vi "CameraManager.vi"(0 "Queue in":refnum<queue>, 2 "Save Setting":T5, 3 "Cluster In":T4={"Camera Mode"=FALSE, "顯示準星"=FALSE, "準星顏色"=65469}, 5 "Camera Manager Data":T3={"Camera Index"=0.0, "Exposure Time"=2800.0, "Image"=refnum, "Save Img Path"=path "C:/Users/MyUser/Pictures", "error out"={"status"=FALSE, "code"=0, "source"=""}, "Specific Parameter"={"Parameter Name"="", "Parameter Value"=""}, "Image Info"={"Height"=0.0, "Width"=0.0, "Channels"=0.0}}, 8 "Select Case":string, 11 "Pic Path":path=path "C:/Users/DavidHsu/OneDrive - PlayNitride/L0_230912/pic/key_pic/20x_2040_rf_k31l.bmp") -> (9 "save img path":path, 14 "Queue out":refnum<queue>, 16 "Initial Status":bool, 17 "Version Info":string, 18 "Camera Count(Output)":i32, 19 "Camera Manager Data Output":T3={"Camera Index"=0.0, "Exposure Time"=2800.0, "Image"=refnum, "Save Img Path"=path "C:/Users/MyUser/Pictures", "error out"={"status"=FALSE, "code"=0, "source"=""}, "Specific Parameter"={"Parameter Name"="", "Parameter Value"=""}, "Image Info"={"Height"=0.0, "Width"=0.0, "Channels"=0.0}})   [LabVIEW 2017, in "PlayNitrideCameraComponet1010_4.lvlib"]
uses:
  <userlib>/PlayNitrideCameraComponet1010_4/PlayNitrideCameraComponet1010_4.lvlib
  <vilib>/vision/Image Controls.llb/IMAQ Image.ctl
  <userlib>/PlayNitrideCameraComponet1010_4/cam_Global.vi
  <resource>/objmgr/IMAQImage.rc
panel:
  out "Camera Mode":bool
  out "Version":string
  in  "Image Info":T1
  out "Camera Count":i32
  out "Initial Success":bool
  out "Stop":bool
  # "中間內部變數 如果有需求可以拉出接口"
  # "Input"
  # "Output"
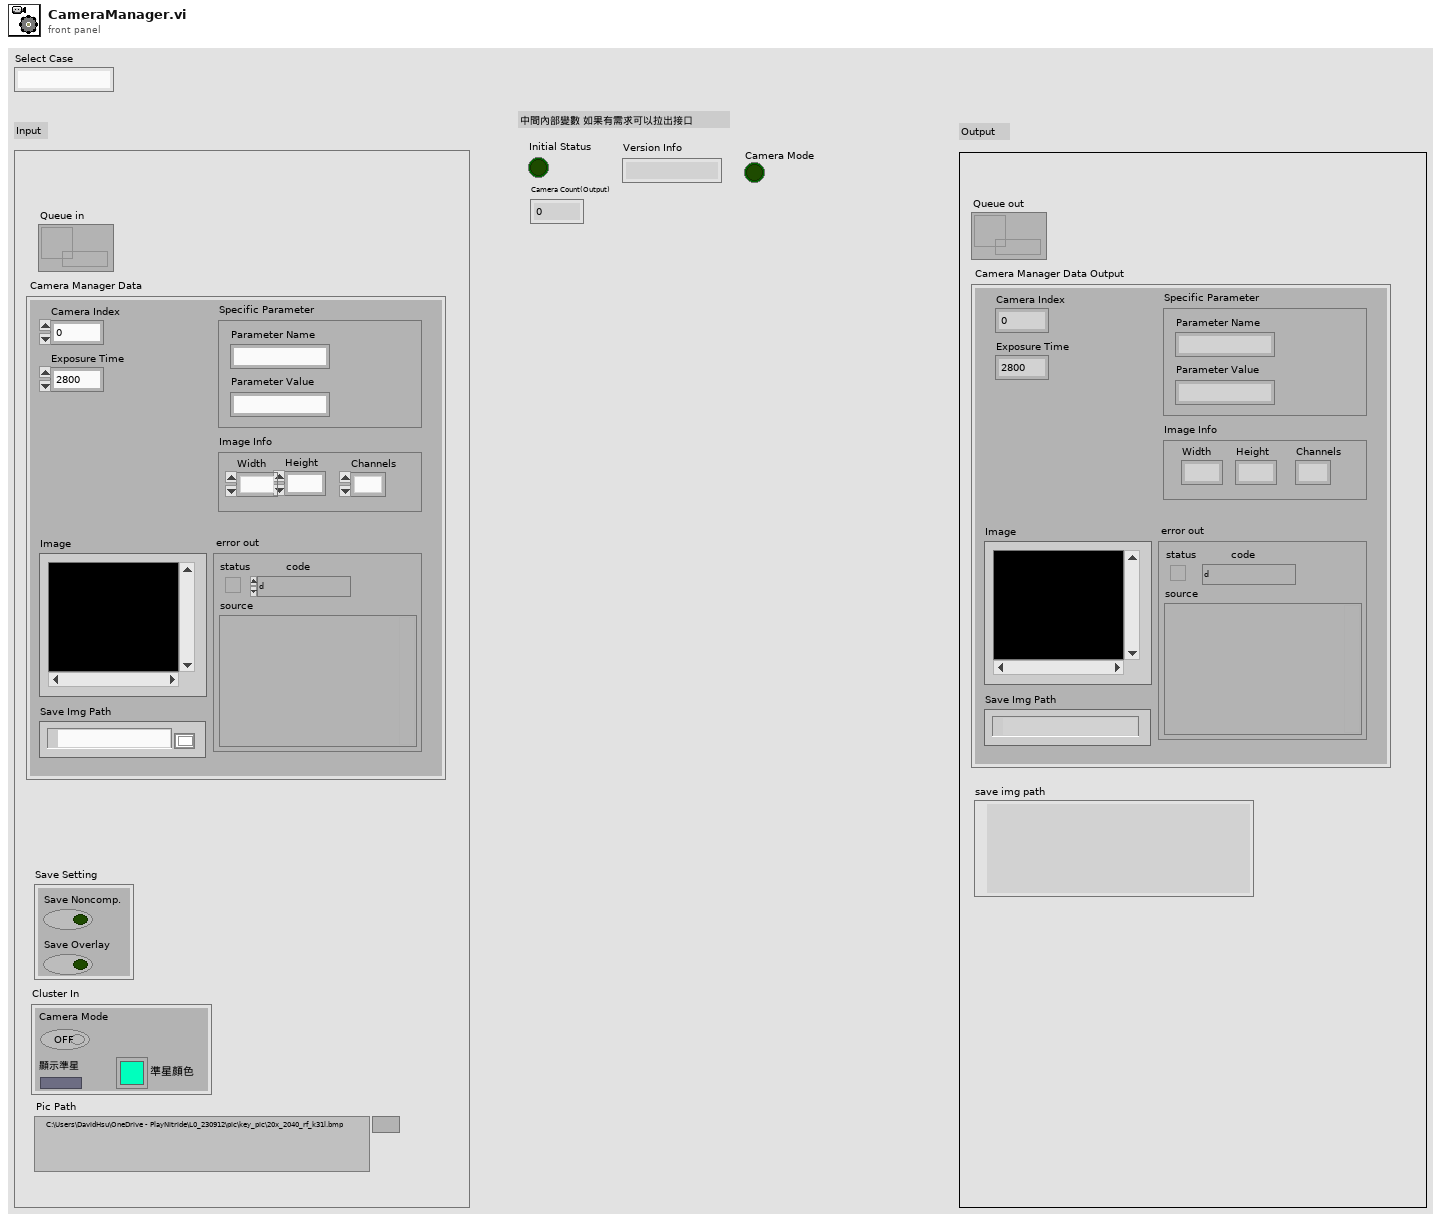
[diagram p1: front panel]
types:
  T1 = cluster{"Height":dbl, "Width":dbl, "Channels":dbl}
  T2 = typedef "IMAQ Image.ctl" = refnum<image>
  T3 = cluster{"Camera Index":dbl, "Exposure Time":dbl, "Image":T2, "Save Img Path":path, "error out":errorcluster, "Specific Parameter":cluster{"Parameter Name":string, "Parameter Value":string}, "Image Info":cluster{"Height":dbl, "Width":dbl, "Channels":dbl}}
  T4 = cluster{"Camera Mode":bool, "顯示準星":bool, "準星顏色":u32}
  T5 = cluster{"Save Noncomp.":bool, "Save Overlay":bool}
  T6 = typedef "Image Type" = u32
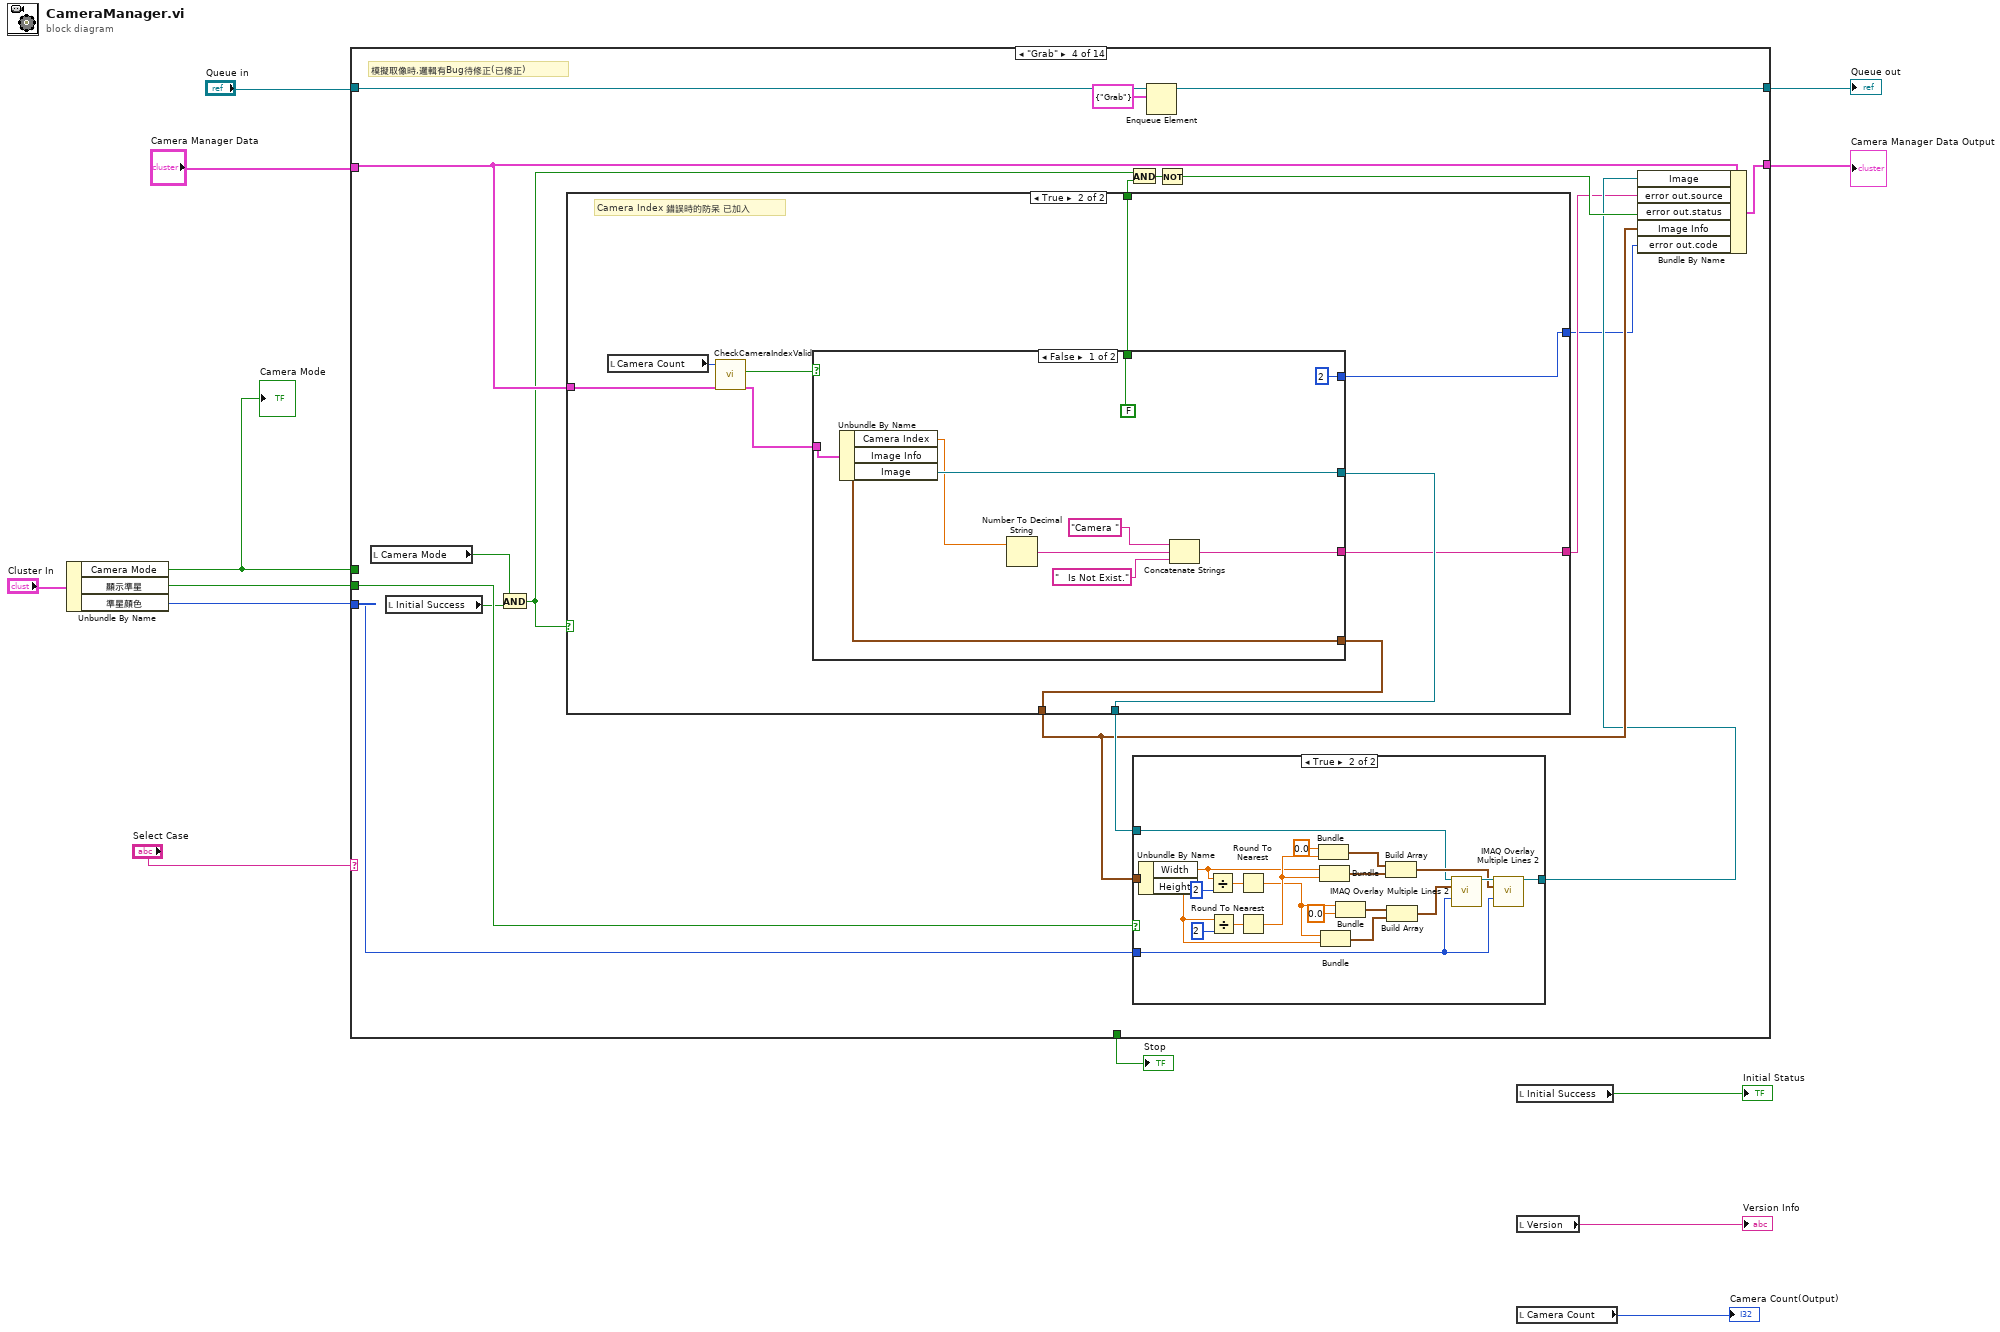
[diagram p0: block diagram]
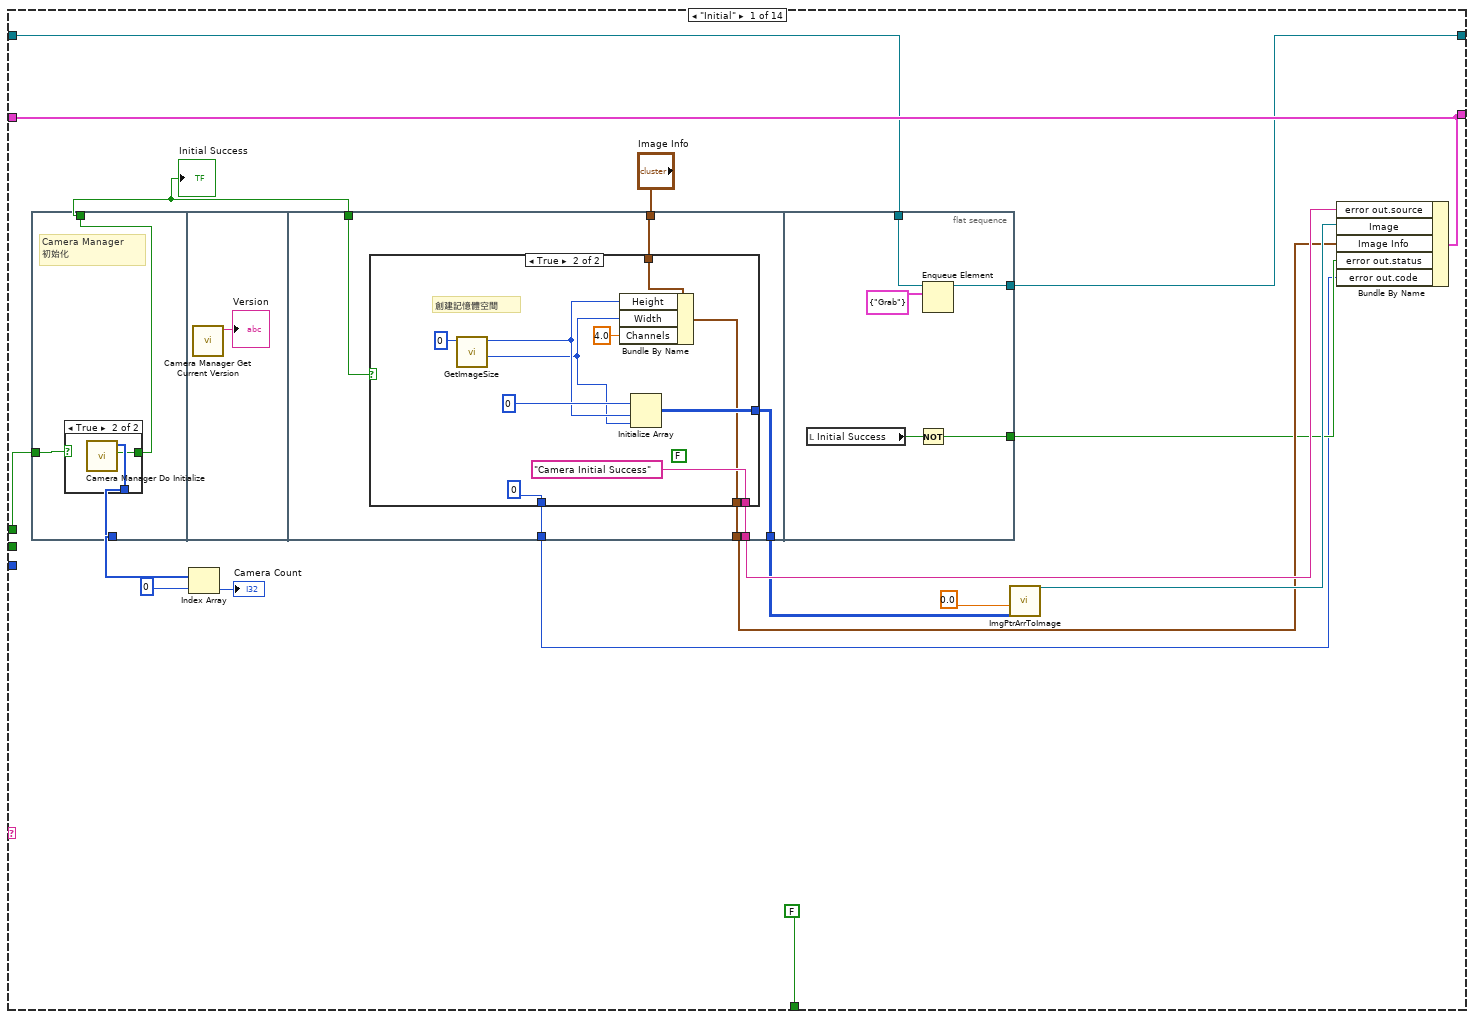
[diagram p2: hidden frame]
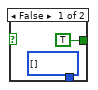
[diagram p3: hidden frame]
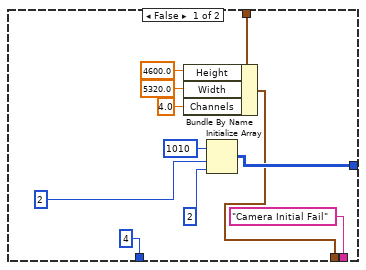
[diagram p4: hidden frame]
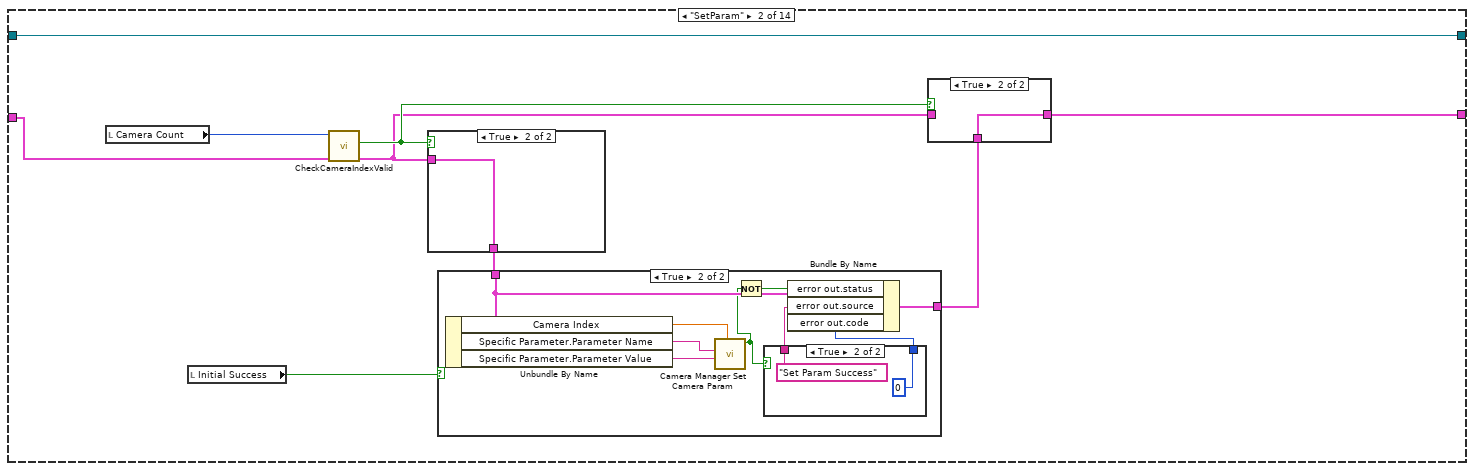
[diagram p5: hidden frame]
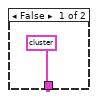
[diagram p7: hidden frame]
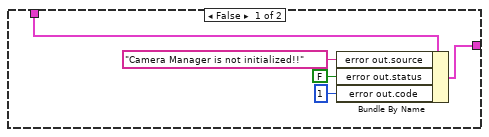
[diagram p8: hidden frame]
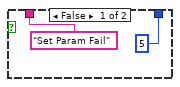
[diagram p9: hidden frame]
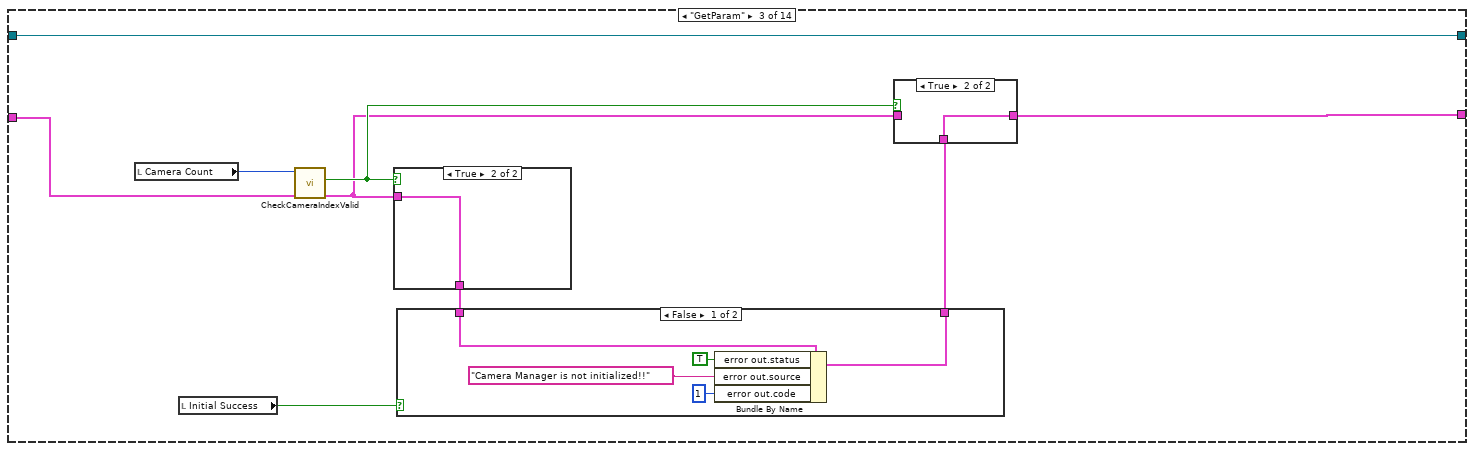
[diagram p10: hidden frame]
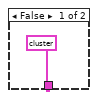
[diagram p12: hidden frame]
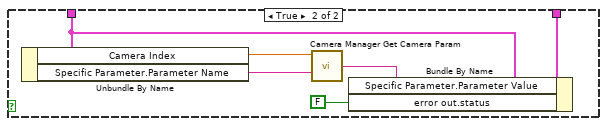
[diagram p13: hidden frame]
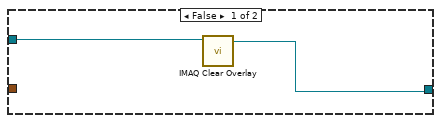
[diagram p14: hidden frame]
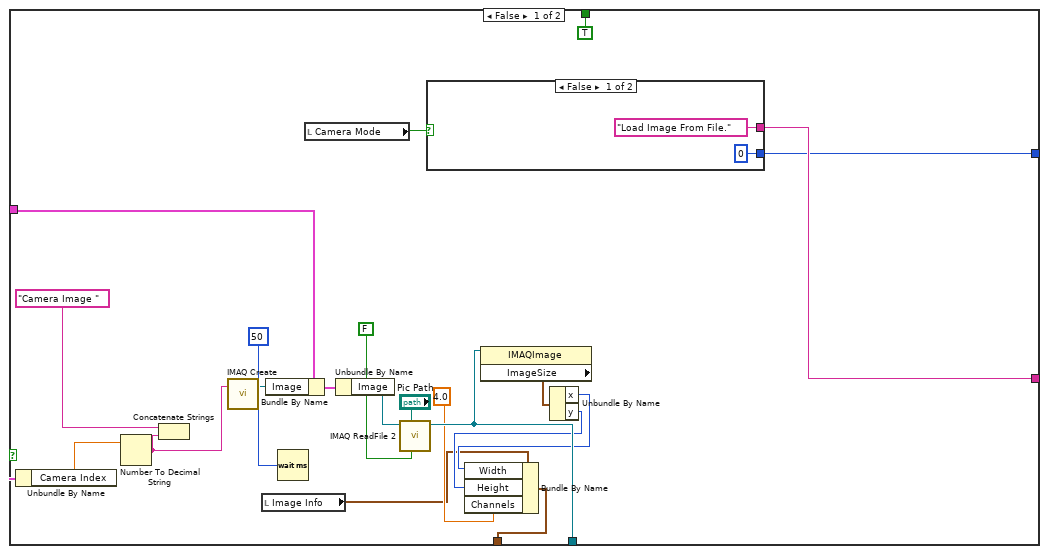
[diagram p15: hidden frame]
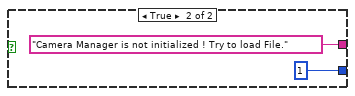
[diagram p16: hidden frame]
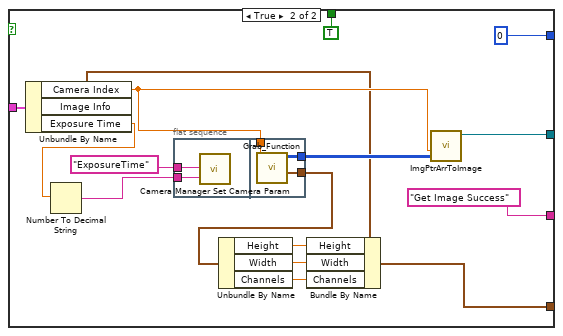
[diagram p17: hidden frame]
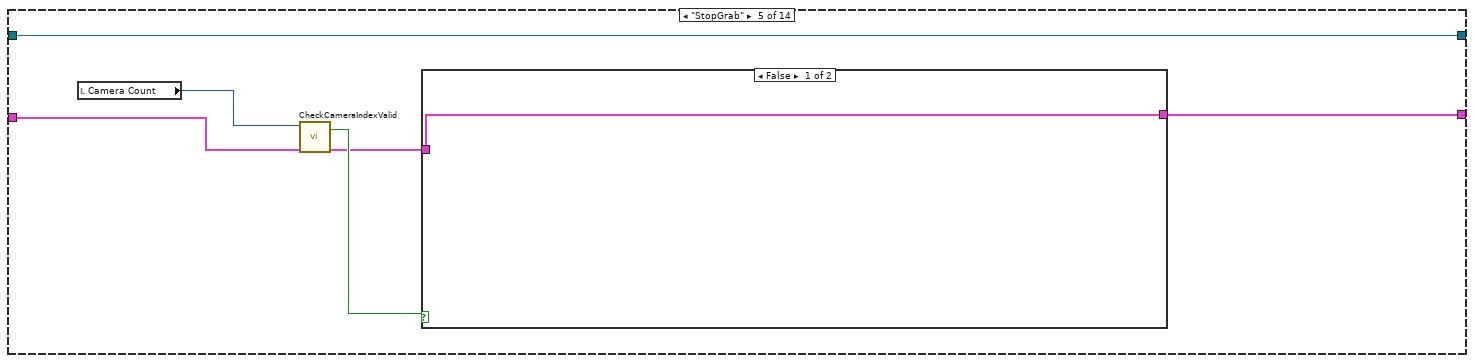
[diagram p18: hidden frame]
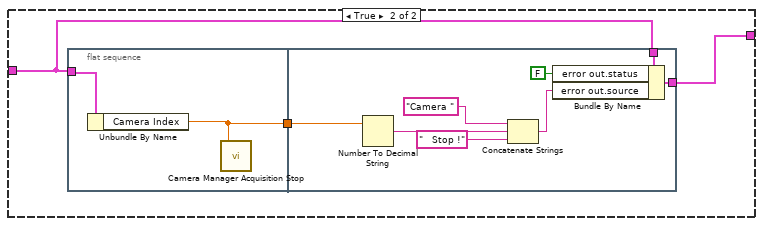
[diagram p19: hidden frame]
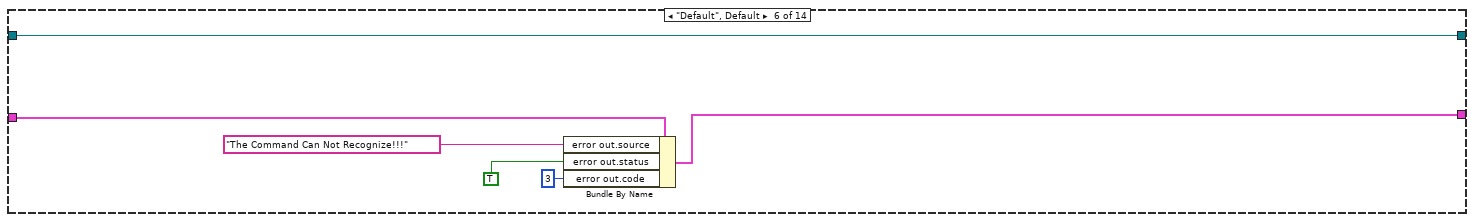
[diagram p20: hidden frame]
diagram:
  n1 = Unbundle By Name("Cluster In") -> ("Camera Mode"=w8:bool, "顯示準星"=w7:bool, "準星顏色"=w6:u32)
  "Camera Mode" <- w8
  n2 = case shown="\"Grab\"" "Select Case" {
    tunnel: "Queue in" -> [w18 w79 w110 w135 w237 w257 w277 w306 w337 w361 w368 w389 w400 w405]
    tunnel: [FALSE _ _ _ _ _ _ _ _ _ _ TRUE _ _] -> w13
    tunnel: [w17 w79 w110 w132 w237 w257 w277 w306 w337 w361 w368 w389 w400 w405] -> w11
    tunnel: [w28 w71 w105 w143 w232 w254 w258 w285 w310 w341 w366 w387 w397 w403] -> w4
    tunnel: "Camera Manager Data" -> [w28 w74 w107 w138 w233 w255 w258 w285 w310 w341 w367 w388 w398 w404]
    tunnel: w8 -> [w16 _ _ _ _ _ _ _ _ _ _ _ _ _]
    tunnel: w7 -> [_ _ _ w141 _ _ _ _ _ _ _ _ _ _]
    tunnel: w6 -> [_ _ _ w142 _ _ _ _ _ _ _ _ _ _]
    frame "Initial" {
      (unwired) FALSE
      n3 = flat-sequence {
        tunnel: [w31] -> w21
        tunnel: [w32] -> w30
        tunnel: w16 -> [w33]
        tunnel: w21 -> [w44]
        tunnel: [w43] -> w26
        tunnel: [w42] -> w27
        tunnel: [w41] -> w23
        tunnel: "Image Info" -> [w40]
        tunnel: [w39] -> w14
        tunnel: [w70] -> w22
        tunnel: w18 -> [w68]
        tunnel: [w67] -> w17
        frame #0 {
          # "Camera Manager \n初始化"
          n4 = case shown="True" w33 {
            tunnel: [i32[] [] ("CameraCount") w37] -> w32
            tunnel: [TRUE ("function return") w36] -> w31
            frame False {
            }
            frame True {
              n5 = call <userlib>:"Camera Manager Do Initialize.vi"() -> ("function return"=w36:bool, "CameraCount"=w37:i32[])  [unwired: 9 in, 1 out]
            }
          }
        }
        frame #1 {
          n6 = call <userlib>:"Camera Manager Get Current Version.vi"() -> ("function return"=→"Version":string)  [unwired: 10 in, 1 out]
        }
        frame #2 {
          n7 = case shown="True" w44 {
            tunnel: [w55 w64] -> w43
            tunnel: ["Camera Initial Fail" ("error out.source") "Camera Initial Success" ("error out.source")] -> w42
            tunnel: [w49 w60] -> w41
            tunnel: w40 -> [w50 w62]
            tunnel: [4 0] -> w39
            frame False {
              n8 = Bundle By Name(cluster=w50, "Height"=4600.0, "Width"=5320.0, "Channels"=4.0) -> (w49:T1)
              n9 = Initialize Array(u32 1010 ("element"), 2 ("dimension size"), 2 ("dimension size")) -> (w55:u32[][])
            }
            frame True {
              # "創建記憶體空間"
              n10 = call <userlib>:"GetImageSize.vi"("cameraId"=0) -> ("Width"=w57:i32, "Height"=w58:i32)  [unwired: 9 in]
              n11 = Bundle By Name(cluster=w62, "Height"=w58, "Width"=w57, "Channels"=4.0) -> (w60:T1)
              n12 = Initialize Array(u32 0 ("unsigned 32bit integer"), w58, w57) -> (w64:u32[][])
            }
          }
        }
        frame #3 {
          n13 = local read "Initial Success"() -> (w69:bool)
          n14 = Not(x=w69) -> (.not. x?=w70:bool)
          n15 = Enqueue Element(queue=w68, element=cluster{"State":string} {"State"="Grab"}) -> (queue out=w67:refnum<queue>)  [unwired: 2 in, 2 out]
        }
      }
      n16 = Index Array(array=w30, index=0) -> (element=→"Camera Count":i32)
      n17 = call <userlib>:"ImgPtrArrToImage.vi"("CameraIndex"=0.0, "Image Pixels (U32)"=w26) -> ("image out"=w25:T2)  [unwired: 8 in, 1 out]
      n18 = Bundle By Name(cluster=w28, "error out.source"=w27, "Image"=w25, "Image Info"=w23, "error out.status"=w22, "error out.code"=w14) -> ()  [unwired: 1 out]
      "Initial Success" <- w21
    }
    frame "SetParam" {
      n19 = local read "Camera Count"() -> (w75:i32)
      n20 = local read "Initial Success"() -> (w78:bool)
      n21 = call <userlib>:"CheckCameraIndexValid.vi"("Camera Manager Data"=w74, "CameraCount"=w75) -> ("Camera Manager Data Out"=w76:T3, "IsValidIndex"=w77:bool)  [unwired: 8 in]
      n22 = case shown="True" w77 {
        tunnel: [T3 {"Camera Index"=0.0, "Exposure Time"=0.0, "Image"=refnum, "Save Img Path"=path "", "error out"={"status"=FALSE, "code"=0, "source"=""}, "Specific Parameter"={"Parameter Name"="", "Parameter Value"=""}, "Image Info"={"Height"=0.0, "Width"=0.0, "Channels"=0.0}} ("Camera Manager Data Out") w83] -> w73
        tunnel: w76 -> [_ w83]
        frame False {
        }
        frame True {
        }
      }
      n23 = case shown="True" w78 {
        tunnel: w73 -> [w88 w96]
        tunnel: [w87 w97] -> w72
        frame False {
          n24 = Bundle By Name(cluster=w88, "error out.source"="Camera Manager is not initialized!!", "error out.status"=FALSE, "error out.code"=1) -> (w87:T3)
        }
        frame True {
          n25 = Unbundle By Name(w96) -> ("Camera Index"=w95:dbl, "Specific Parameter.Parameter Name"=w94:string, "Specific Parameter.Parameter Value"=w93:string)
          n26 = call <userlib>:"Camera Manager Set Camera Param.vi"("Value"=w93, "NodeName"=w94, "cameraId"=w95) -> ("function return"=w90:bool)  [unwired: 5 in, 3 out]
          n27 = Not(x=w90) -> (.not. x?=w89:bool)
          n28 = case shown="True" w90 {
            tunnel: ["Set Param Fail" ("error out.source") "Set Param Success" ("error out.source")] -> w92
            tunnel: [5 0] -> w91
            frame False {
            }
            frame True {
            }
          }
          n29 = Bundle By Name(cluster=w96, "error out.status"=w89, "error out.source"=w92, "error out.code"=w91) -> (w97:T3)
        }
      }
      n30 = case shown="True" w77 {
        tunnel: [w80 w81] -> w71
        tunnel: w72 -> [_ w81]
        tunnel: w76 -> [w80 _]
        frame False {
        }
        frame True {
        }
      }
    }
    frame "GetParam" {
      n31 = local read "Camera Count"() -> (w108:i32)
      n32 = local read "Initial Success"() -> (w109:bool)
      n33 = call <userlib>:"CheckCameraIndexValid.vi"("Camera Manager Data"=w107, "CameraCount"=w108) -> ("Camera Manager Data Out"=w102:T3, "IsValidIndex"=w103:bool)  [unwired: 8 in]
      n34 = case shown="True" w103 {
        tunnel: [T3 {"Camera Index"=0.0, "Exposure Time"=0.0, "Image"=refnum, "Save Img Path"=path "", "error out"={"status"=FALSE, "code"=0, "source"=""}, "Specific Parameter"={"Parameter Name"="", "Parameter Value"=""}, "Image Info"={"Height"=0.0, "Width"=0.0, "Channels"=0.0}} ("Camera Manager Data Out") w114] -> w106
        tunnel: w102 -> [_ w114]
        frame False {
        }
        frame True {
        }
      }
      n35 = case shown="False" w109 {
        tunnel: w106 -> [w119 w125]
        tunnel: [w118 w124] -> w104
        frame False {
          n36 = Bundle By Name(cluster=w119, "error out.status"=TRUE, "error out.source"="Camera Manager is not initialized!!", "error out.code"=1) -> (w118:T3)
        }
        frame True {
          n37 = Unbundle By Name(w125) -> ("Camera Index"=w120:dbl, "Specific Parameter.Parameter Name"=w121:string)
          n38 = call <userlib>:"Camera Manager Get Camera Param.vi"("NodeName"=w121, "cameraId"=w120) -> ("Value out"=w122:string)  [unwired: 7 in, 2 out]
          n39 = Bundle By Name(cluster=w125, "Specific Parameter.Parameter Value"=w122, "error out.status"=FALSE) -> (w124:T3)
        }
      }
      n40 = case shown="True" w103 {
        tunnel: [w111 w112] -> w105
        tunnel: w104 -> [_ w112]
        tunnel: w102 -> [w111 _]
        frame False {
        }
        frame True {
        }
      }
    }
    frame "Grab" {
      # "模擬取像時,邏輯有Bug待修正(已修正)"
      n41 = local read "Camera Mode"() -> (w134:bool)
      n42 = local read "Initial Success"() -> (w136:bool)
      n43 = And(x=w134, y=w136) -> (x .and. y?=w129:bool)
      n44 = case shown="True" w129 {
        tunnel: [w169 w195] -> w130
        tunnel: [w180 w197] -> w137
        tunnel: [w185 w196] -> w140
        tunnel: w138 -> [w174 w194]
        tunnel: [TRUE ("y") w193] -> w127
        tunnel: [w167 w192] -> w126
        frame False {
          n45 = Unbundle By Name(w174) -> ("Camera Index"=w173:dbl)
          n46 = Number To Decimal String(number=w173) -> (decimal integer string=w172:string)  [unwired: 1 in]
          n47 = Concatenate Strings("Camera Image " ("string"), w172) -> ()  [unwired: 1 out]
          n48 = call "IMAQ Create"("Image Name"=w172) -> ("New Image"=w176:T2)  [unwired: 4 in, 1 out]
          n49 = local read "Image Info"() -> (w179:T1)
          n50 = Bundle By Name(cluster=w174, "Image"=w176) -> (w178:T3)
          n51 = Wait (ms)(milliseconds to wait=u32 50) -> ()  [unwired: 1 out]
          n52 = local read "Camera Mode"() -> (w170:bool)
          n53 = Unbundle By Name(w178) -> ("Image"=w177:T2)
          n54 = call "IMAQ ReadFile 2"("Use File Path Image Type"=FALSE, "File Path"="Pic Path", "Image"=w177) -> ("Image Out"=w185:T2)  [unwired: 4 in, 4 out]
          n55 = case shown="False" w170 {
            tunnel: ["Load Image From File." ("error out.source") "Camera Manager is not initialized ! Try to load File." ("error out.source")] -> w169
            tunnel: [0 1] -> w167
            frame False {
            }
            frame True {
            }
          }
          n56 = property class="IMAQImage"(reference=w185) -> ("ImageSize"=w184:cluster{"x":i32, "y":i32})  [unwired: 1 in, 2 out]
          n57 = Unbundle By Name(w184) -> ("x"=w182:i32, "y"=w181:i32)
          n58 = Bundle By Name(cluster=w179, "Width"=w182, "Height"=w181, "Channels"=4.0) -> (w180:T1)
        }
        frame True {
          # "Camera Index 錯誤時的防呆 已加入"
          n59 = local read "Camera Count"() -> (w200:i32)
          n60 = call <userlib>:"CheckCameraIndexValid.vi"("Camera Manager Data"=w194, "CameraCount"=w200) -> ("Camera Manager Data Out"=w198:T3, "IsValidIndex"=w199:bool)  [unwired: 8 in]
          n61 = case shown="False" w199 {
            tunnel: w198 -> [w210 w217]
            tunnel: [w203 "Get Image Success" ("error out.source")] -> w195
            tunnel: [w206 w215] -> w197
            tunnel: [w205 w213] -> w196
            tunnel: [FALSE ("y") TRUE ("y")] -> w193
            tunnel: [2 0] -> w192
            frame False {
              n62 = Unbundle By Name(w210) -> ("Camera Index"=w202:dbl, "Image Info"=w206:T1, "Image"=w205:T2)
              n63 = Number To Decimal String(number=w202) -> (decimal integer string=w209:string)  [unwired: 1 in]
              n64 = Concatenate Strings("Camera " ("string"), w209, "   Is Not Exist." ("string")) -> (w203:string)
            }
            frame True {
              n65 = Unbundle By Name(w217) -> ("Camera Index"=w226:dbl, "Image Info"=w219:T1, "Exposure Time"=w214:dbl)
              n66 = Number To Decimal String(number=w214) -> (decimal integer string=w225:string)  [unwired: 1 in]
              n67 = flat-sequence {
                tunnel: "ExposureTime" ("NodeName") -> [w228]
                tunnel: w225 -> [w227]
                tunnel: [w231] -> w223
                tunnel: [w230] -> w224
                tunnel: w226 -> [w229]
                frame #0 {
                  n68 = call <userlib>:"Camera Manager Set Camera Param.vi"("Value"=w227, "NodeName"=w228) -> ()  [unwired: 6 in, 4 out]
                }
                frame #1 {
                  n69 = call <userlib>:"Grab_Function.vi"("cameraId"=w229) -> ("output cluster"=w231:T1, "imgPtr"=w230:i32[][])  [unwired: 7 in]
                }
              }
              n70 = Unbundle By Name(w223) -> ("Height"=w220:dbl, "Width"=w221:dbl, "Channels"=w222:dbl)
              n71 = Bundle By Name(cluster=w219, "Height"=w220, "Width"=w221, "Channels"=w222) -> (w215:T1)
              n72 = call <userlib>:"ImgPtrArrToImage.vi"("CameraIndex"=w226, "Image Pixels (U32)"=w224) -> ("image out"=w213:T2)  [unwired: 8 in, 1 out]
            }
          }
        }
      }
      n73 = And(x=w129, y=w127) -> (x .and. y?=w128:bool)
      n74 = case shown="True" w141 {
        tunnel: [w145 w165] -> w131
        tunnel: w137 -> [_ w155]
        tunnel: w140 -> [w144 w146]
        tunnel: w142 -> [_ w147]
        frame False {
          n75 = call "IMAQ Clear Overlay"("Image"=w144) -> ("Image Out"=w145:T2)  [unwired: 9 in, 1 out]
        }
        frame True {
          n76 = Unbundle By Name(w155) -> ("Width"=w161:dbl, "Height"=w148:dbl)
          n77 = Divide(x=w161, y=2) -> (x/y=w156:dbl)
          n78 = Divide(x=w148, y=2) -> (x/y=w157:dbl)
          n79 = Round To Nearest(number=w156) -> (nearest integer value=w162:dbl)
          n80 = Round To Nearest(number=w157) -> (nearest integer value=w164:dbl)
          n81 = Bundle("X"=0.0, w164) -> (w163:cluster{"X":dbl, dbl})  [unwired: 1 in]
          n82 = Bundle("Width"=w161, w164) -> (w160:cluster{"Width":dbl, dbl})  [unwired: 1 in]
          n83 = Bundle(w162, "Height"=w148) -> (w159:cluster{dbl, "Height":dbl})  [unwired: 1 in]
          n84 = Bundle(w162, "X"=0.0) -> (w158:cluster{dbl, "X":dbl})  [unwired: 1 in]
          n85 = Build Array(w163, w160) -> (w150:cluster{"Width":dbl, dbl}[])
          n86 = Build Array(w158, w159) -> (w149:cluster{dbl, "Height":dbl}[])
          n87 = call "IMAQ Overlay Multiple Lines 2"("Image"=w146, "Line End Points"=w149, "Color"=w147) -> ("Image Out"=w166:T2)  [unwired: 11 in, 1 out]
          n88 = call "IMAQ Overlay Multiple Lines 2"("Image"=w166, "Line End Points"=w150, "Color"=w147) -> ("Image Out"=w165:T2)  [unwired: 11 in, 1 out]
        }
      }
      n89 = Enqueue Element(queue=w135, element=cluster{"State":string} {"State"="Grab"}) -> (queue out=w132:refnum<queue>)  [unwired: 2 in, 2 out]
      n90 = Not(x=w128) -> (.not. x?=w139:bool)
      n91 = Bundle By Name(cluster=w138, "Image"=w131, "error out.source"=w130, "error out.status"=w139, "Image Info"=w137, "error out.code"=w126) -> (w143:T3)
    }
    frame "StopGrab" {
      n92 = local read "Camera Count"() -> (w236:i32)
      n93 = call <userlib>:"CheckCameraIndexValid.vi"("Camera Manager Data"=w233, "CameraCount"=w236) -> ("Camera Manager Data Out"=w234:T3, "IsValidIndex"=w235:bool)  [unwired: 8 in]
      n94 = case shown="False" w235 {
        tunnel: w234 -> [w238 w239]
        tunnel: [w238 w241] -> w232
        frame False {
        }
        frame True {
          n95 = flat-sequence {
            tunnel: w239 -> [w243]
            tunnel: [w242] -> w240
            tunnel: w239 -> [w249]
            tunnel: [w245] -> w241
            tunnel: w240 -> [w244]
            frame #0 {
              n96 = Unbundle By Name(w243) -> ("Camera Index"=w242:dbl)
              n97 = call <userlib>:"Camera Manager Acquisition Stop.vi"("cameraId"=w242) -> ()  [unwired: 10 in, 1 out]
            }
            frame #1 {
              n98 = Number To Decimal String(number=w244) -> (decimal integer string=w250:string)  [unwired: 1 in]
              n99 = Concatenate Strings("Camera " ("string"), w250, "   Stop !" ("string")) -> (w251:string)
              n100 = Bundle By Name(cluster=w249, "error out.status"=FALSE, "error out.source"=w251) -> (w245:T3)
            }
          }
        }
      }
    }
    frame "Default", Default {
      n101 = Bundle By Name(cluster=w255, "error out.source"="The Command Can Not Recognize!!!", "error out.status"=TRUE, "error out.code"=3) -> (w254:T3)
    }
    frame "Save Img" {
      # "這邊完全照抄 Kernel_Camera.vi 的內容"
      n102 = Unbundle By Name(w258) -> ("Save Img Path"=w272:path, "Image"=w265:T2)
      n103 = Get Date/Time In Seconds() -> (seconds since 1Jan1904=w271:timestamp)
      n104 = Unbundle By Name("Save Setting") -> ("Save Noncomp."=w262:bool, "Save Overlay"=w267:bool)
      n105 = Format Date/Time String(time format string (%c)="%Y%m%d_%H%M%S", seconds (now)=w271) -> (date/time string=w269:string)  [unwired: 1 in]
      n106 = global read "cam_Global.vi" "img_suffix"() -> (w260:string)
      n107 = Path To String(path=w272) -> (string=w275:string)
      n108 = case shown="True" w267 {
        tunnel: [w282 w283] -> w266
        tunnel: w265 -> [w282 w284]
        frame False {
        }
        frame True {
          n109 = call "IMAQ Merge Overlay"("Image Src"=w284) -> ("Image Dst Out"=w283:T2)  [unwired: 9 in, 1 out]
        }
      }
      n110 = Select(t=".bmp" ("string"), s=w262, f=".jpeg" ("string")) -> (s? t:f=w259:string)
      n111 = Concatenate Strings(w275, "\\" ("string"), w269, "_" ("string"), w260, w259) -> (w273:string)
      n112 = String To Path(string=w273) -> (path=w274:path)
      "save img path" <- w274
      n113 = case shown="False" w262 {
        tunnel: w274 -> [w279 w281]
        tunnel: w266 -> [w278 w280]
        frame True {
          n114 = call-poly "IMAQ Write File 2"("File Path"=w279, "Image"=w278) -> ()  [unwired: 8 in, 2 out]
        }
        frame False {
          n115 = call-poly "IMAQ Write File 2"("File Path"=w281, "Image"=w280) -> ()  [unwired: 8 in, 2 out]
        }
      }
    }
    frame "Save Failure" {
      w291 = 0 items=["Desktop"=0, "Personal Documents"=5, "AppData"=26, "Local AppData"=28, "Common AppData"=35, "Program Files"=38, "Program Files Common"=43, "Common Documents"=46] ("Requested Path")
      # "這邊完全照抄 Kernel_Camera.vi 的內容"
      n116 = Unbundle By Name(w285) -> ("Image"=w302:T2)  [unwired: 1 out]
      n117 = global read "cam_Global.vi" "failure_suffix"() -> (w298:string)
      n118 = call "Get Windows File Locations.vi"("Requested Path"=w291) -> ("path"=w303:path)  [unwired: 9 in, 1 out]
      n119 = Get Date/Time In Seconds() -> (seconds since 1Jan1904=w292:timestamp)
      n120 = Build Path(base path=w303, name or relative path="program\\img_failure") -> (appended path=w294:path)
      n121 = Format Date/Time String(time format string (%c)="%Y%m%d_%H%M%S", seconds (now)=w292) -> (date/time string=w293:string)  [unwired: 1 in]
      n122 = call <vilib>:"Check if File or Folder Exists.vi"("path"=w294) -> ("file or folder exists?"=w296:bool, "dup path"=w295:path)  [unwired: 8 in, 1 out]
      n123 = case shown="False" w296 {
        tunnel: w295 -> [w307 w309]
        tunnel: [w307 w308] -> w297
        frame True {
        }
        frame False {
          n124 = Create Folder(path (use dialog)=w309) -> (created path=w308:path)  [unwired: 2 in, 2 out]
        }
      }
      n125 = Concatenate Strings("\\" ("string"), w293, "_" ("string"), w298, ".bmp" ("string")) -> (w301:string)
      n126 = Path To String(path=w297) -> (string=w300:string)
      n127 = Concatenate Strings(w300, w301) -> (w299:string)
      n128 = String To Path(string=w299) -> (path=w304:path)
      n129 = call-poly "IMAQ Write File 2"("File Path"=w304, "Image"=w302) -> ()  [unwired: 8 in, 2 out]
      n130 = call <userlib>:"Check valid path.vi"("Path"=w304) -> ("valid path"=w305:bool)  [unwired: 10 in]
      n131 = case shown="False" w305 {
        frame False {
          (unwired) "" ("Input")
        }
        frame True {
        }
      }
    }
    frame "Save Crop Pattern" {
      w317 = T6 4 items=["Grayscale (U8)", "Grayscale (I16)", "Grayscale (SGL)", "Complex (CSG)", "RGB (U32)", "HSL (U32)", "RGB (U64)", "Grayscale (U16)"] ("Image Type")
      w316 = 0 items=["Desktop"=0, "Personal Documents"=5, "AppData"=26, "Local AppData"=28, "Common AppData"=35, "Program Files"=38, "Program Files Common"=43, "Common Documents"=46] ("Requested Path")
      # "這邊完全照抄 Kernel_Camera.vi 的內容"
      n132 = call "Get Windows File Locations.vi"("Requested Path"=w316) -> ("path"=w327:path)  [unwired: 9 in, 1 out]
      n133 = Unbundle By Name(w310) -> ("Image"=w330:T2)  [unwired: 1 out]
      n134 = Build Path(base path=w327, name or relative path="program\\Pattern") -> (appended path=w320:path)
      n135 = global read "cam_Global.vi" "Global Rectangle"() -> (w334:i32[])
      n136 = call <vilib>:"Check if File or Folder Exists.vi"("path"=w320) -> ("file or folder exists?"=w322:bool, "dup path"=w321:path)  [unwired: 8 in, 1 out]
      n137 = global read "cam_Global.vi" "crop_suffix"() -> (w335:string)
      n138 = call "IMAQ Create"("Image Name"="Cam1Crop", "Image Type"=w317) -> ("New Image"=w332:T2)  [unwired: 3 in, 1 out]
      n139 = Get Date/Time In Seconds() -> (seconds since 1Jan1904=w319:timestamp)
      n140 = case shown="False" w322 {
        tunnel: w321 -> [w338 w340]
        tunnel: [w338 w339] -> w323
        frame True {
        }
        frame False {
          n141 = Create Folder(path (use dialog)=w340) -> (created path=w339:path)  [unwired: 2 in, 2 out]
        }
      }
      n142 = Format Date/Time String(time format string (%c)="%Y%m%d_%H%M%S", seconds (now)=w319) -> (date/time string=w336:string)  [unwired: 1 in]
      n143 = call "IMAQ ColorImageToArray"("Optional Rectangle"=w334, "Image"=w330) -> ("Image Pixels (U32)"=w329:u32[][])  [unwired: 2 in, 2 out]
      n144 = Path To String(path=w323) -> (string=w325:string)
      n145 = call "IMAQ ArrayToColorImage"("Image Pixels (U32)"=w329, "Image"=w332) -> ("Image Out"=w331:T2)  [unwired: 3 in, 1 out]
      n146 = Concatenate Strings("\\" ("string"), w335, "_" ("string"), w336, ".bmp" ("string")) -> (w326:string)
      n147 = Concatenate Strings(w325, w326) -> (w324:string)
      n148 = String To Path(string=w324) -> (path=w328:path)
      n149 = call-poly "IMAQ Write File 2"("File Path"=w328, "Image"=w331) -> ("Image Out (duplicate)"=w333:T2)  [unwired: 8 in, 1 out]
      n150 = call "IMAQ Dispose"("Image"=w333) -> ()  [unwired: 5 in, 1 out]
    }
    frame "Save Toggle" {
      w347 = 0 items=["Desktop"=0, "Personal Documents"=5, "AppData"=26, "Local AppData"=28, "Common AppData"=35, "Program Files"=38, "Program Files Common"=43, "Common Documents"=46] ("Requested Path")
      # "這邊完全照抄 Kernel_Camera.vi 的內容"
      n151 = call "Get Windows File Locations.vi"("Requested Path"=w347) -> ("path"=w359:path)  [unwired: 9 in, 1 out]
      n152 = Unbundle By Name(w341) -> ("Image"=w360:T2)  [unwired: 1 out]
      n153 = Build Path(base path=w359, name or relative path="program\\img_manual_save") -> (appended path=w351:path)
      n154 = global read "cam_Global.vi" "img_suffix"() -> (w355:string)
      n155 = call <vilib>:"Check if File or Folder Exists.vi"("path"=w351) -> ("file or folder exists?"=w353:bool, "dup path"=w352:path)  [unwired: 8 in, 1 out]
      n156 = Get Date/Time In Seconds() -> (seconds since 1Jan1904=w349:timestamp)
      n157 = Format Date/Time String(time format string (%c)="%Y%m%d_%H%M%S", seconds (now)=w349) -> (date/time string=w350:string)  [unwired: 1 in]
      n158 = case shown="False" w353 {
        tunnel: w352 -> [w362 w364]
        tunnel: [w362 w363] -> w354
        frame True {
        }
        frame False {
          n159 = Create Folder(path (use dialog)=w364) -> (created path=w363:path)  [unwired: 2 in, 2 out]
        }
      }
      n160 = Path To String(path=w354) -> (string=w356:string)
      n161 = Concatenate Strings("\\" ("string"), w350, "_" ("string"), w355, ".bmp" ("string")) -> (w358:string)
      n162 = Concatenate Strings(w356, w358) -> (w357:string)
      n163 = String To Path(string=w357) -> (path=w348:path)
      n164 = call-poly "IMAQ Write File 2"("File Path"=w348, "Image"=w360) -> ()  [unwired: 8 in, 2 out]
    }
    frame "Settings" {
      n165 = local read "Initial Success"() -> (w365:bool)
      n166 = case shown="True" w365 {
        tunnel: w367 -> [w372 w380]
        tunnel: [w371 w381] -> w366
        frame False {
          n167 = Bundle By Name(cluster=w372, "error out.source"="Camera Manager is not initialized!!", "error out.status"=FALSE) -> (w371:T3)
        }
        frame True {
          n168 = Unbundle By Name(w380) -> ("Camera Index"=w379:dbl, "Exposure Time"=w376:dbl)
          n169 = Number To Decimal String(number=w376) -> (decimal integer string=w374:string)  [unwired: 1 in]
          n170 = call <userlib>:"Camera Manager Set Camera Param.vi"("Value"=w374, "NodeName"="ExposureTime", "cameraId"=w379) -> ("function return"=w378:bool)  [unwired: 5 in, 3 out]
          n171 = case shown="True" w378 {
            tunnel: ["Set Param Fail" ("error out.source") "Set Param Success" ("error out.source")] -> w377
            tunnel: [5 0] -> w373
            frame False {
            }
            frame True {
            }
          }
          n172 = Bundle By Name(cluster=w380, "error out.source"=w377, "error out.code"=w373) -> (w381:T3)
        }
      }
    }
    frame "Shutdown" {
      n173 = local read "Initial Success"() -> (w386:bool)
      n174 = flat-sequence {
        tunnel: w386 -> [w391]
        tunnel: [w396] -> w387
        tunnel: w388 -> [w395]
        frame #0 {
          n175 = case shown="True" w391 {
            frame False {
            }
            frame True {
              n176 = call <userlib>:"Camera Manager Un Initialize.vi"() -> ()  [unwired: 11 in, 1 out]
            }
          }
        }
        frame #1 {
          n177 = local write "Initial Success"(FALSE ("Initial Success")) -> ()
          n178 = local write "Camera Count"(0 ("Camera Count")) -> ()
        }
        frame #2 {
          n179 = Bundle By Name(cluster=w395, "error out.source"="CameraManager Shut Down Sucess.") -> (w396:T3)
        }
      }
    }
    frame "SaveParameter" {
      n180 = Unbundle By Name(w398) -> ("Camera Index"=w401:dbl)
      n181 = call <userlib>:"Camera Manager Save Param.vi"("cameraId"=w401) -> ("error out"=w399:errorcluster)  [unwired: 10 in]
      n182 = Bundle By Name(cluster=w398, "error out"=w399) -> (w397:T3)
    }
    frame "LoadParameter" {
      n183 = Unbundle By Name(w404) -> ("Camera Index"=w406:dbl)
      n184 = call <userlib>:"Camera Manager Load Param.vi"("cameraId"=w406) -> ("error out"=w402:errorcluster)  [unwired: 10 in]
      n185 = Bundle By Name(cluster=w404, "error out"=w402) -> (w403:T3)
    }
  }
  "Stop" <- w13
  "Queue out" <- w11
  "Camera Manager Data Output" <- w4
  n186 = local read "Initial Success"() -> (→"Initial Status":bool)
  n187 = local read "Version"() -> (→"Version Info":string)
  n188 = local read "Camera Count"() -> (→"Camera Count(Output)":i32)
